vi "Life Support.vi"() -> ()   [LabVIEW 2020]
uses:
  <vilib>/regexp/Match Regular Expression.xnode
panel:
  out "Life Support":u32
  out "CO2":u32
  out "O2":u32
  in  "Input":string="110011110101\n110011100010\n010100011010\n011001100000\n010011011101\n011110111000\n111111000100\n000100010001\n101101010011\n100101101100\n001111011010\n011111111101\n010111000000\n000011101000\n100101010010\n010011000010\n000011000000\n111100110010\n100100101110\n110000110100\n011110010000\n010101000000\n001000110001\n010111000100\n110111010100\n011001110110\n110001001101\n001101010010\n110111110100\n100111110111\n001001110010\n001100011111\n001111110010\n100111000111\n101111100001\n011100001100\n000000000111\n101111110001\n110111001101\n101111011010\n100101001111\n011101111111\n101101010101\n011011111000\n011100101001\n001101010100\n00..."
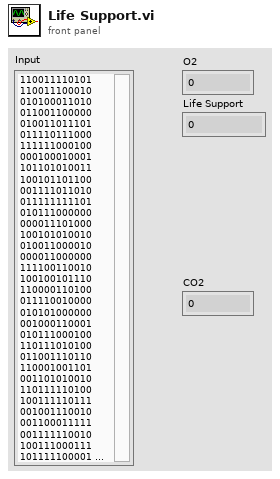
[diagram p1: front panel]
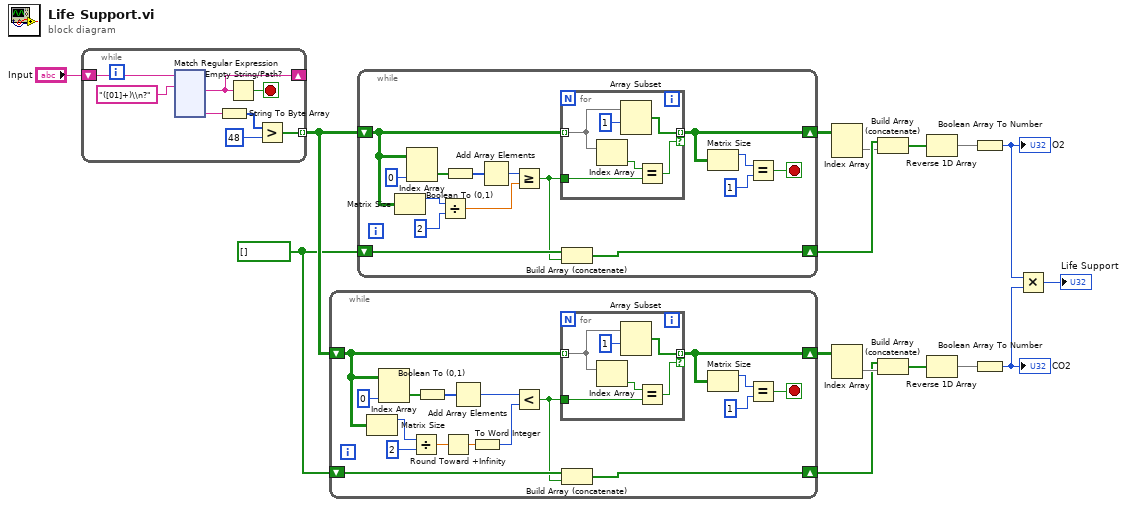
[diagram p0: block diagram]
diagram:
  w4 = bool[] []
  n1 = while {
    shift-right: [w22] -> _
    shift-left: "Input" -> [w24]
    tunnel: [w17] -> w5 mode=indexing
    stop <- w21 stop-if-true
    n2 = xnode "Match Regular Expression"("input string"=w24, "regular expression"="([01]+)\\n?") -> ("after match"=w22:string, "submatch 1"=w20:string)  [unwired: 4 in, 4 out]
    n3 = String To Byte Array(string=w20) -> (unsigned byte array=w19:u8[])
    n4 = Empty String/Path?(string/path=w22) -> (empty?=w21:bool)
    n5 = Greater?(x=w19, y=u8 48) -> (0:w17:bool[])
  }
  n6 = while {
    shift-right: [w150] -> w6
    shift-left: w4 -> [w152]
    shift-right: [w149] -> w7
    shift-left: w5 -> [w153]
    stop <- w147 stop-if-true
    n7 = Matrix Size(0:w153) -> (1:w145:i32)  [unwired: 1 out]
    n8 = Index Array(array=w153, index (col)=0 ("disabled index (col)")) -> (element=w156:bool[])  [unwired: 1 in]
    n9 = Divide(x=w145, y=2) -> (x/y=w143:dbl)
    n10 = Boolean To (0,1)(Boolean=w156) -> (0, 1=w155:i16[])
    n11 = Round Toward +Infinity(x=w143) -> (ceil(x): smallest int >= x=w142:dbl)
    n12 = Add Array Elements(numeric array=w155) -> (sum=w154:i16)
    n13 = To Word Integer(number=w142) -> (16bit integer=w141:i16)
    n14 = Less?(x=w154, y=w141) -> (x < y?=w151:bool)
    n15 = for {
      tunnel: w153 -> [w161] mode=indexing
      tunnel: w151 -> [w163]
      tunnel: [w159] -> w149 mode=indexing if=w158
      n16 = Index Array(array=w161) -> (element=w162:bool)  [unwired: 1 in]
      n17 = Array Subset(array=w161, index=1) -> (w159:bool[])  [unwired: 1 in]
      n18 = Equal?(x=w162, y=w163) -> (x = y?=w158:bool)
    }
    n19 = Build Array (concatenate)(w152, w151) -> (w150:bool[])
    n20 = Matrix Size(0:w149) -> (1:w146:i32)  [unwired: 1 out]
    n21 = Equal?(x=w146, y=1) -> (x = y?=w147:bool)
  }
  n22 = while {
    shift-right: [w171] -> w15
    shift-left: w4 -> [w173]
    shift-right: [w170] -> w14
    shift-left: w5 -> [w174]
    stop <- w168 stop-if-true
    n23 = Matrix Size(0:w174) -> (1:w166:i32)  [unwired: 1 out]
    n24 = Index Array(array=w174, index (col)=0 ("disabled index (col)")) -> (element=w177:bool[])  [unwired: 1 in]
    n25 = Divide(x=w166, y=2) -> (x/y=w164:dbl)
    n26 = Boolean To (0,1)(Boolean=w177) -> (0, 1=w176:i16[])
    n27 = Add Array Elements(numeric array=w176) -> (sum=w175:i16)
    n28 = Greater Or Equal?(x=w175, y=w164) -> (x >= y?=w172:bool)
    n29 = for {
      tunnel: w174 -> [w182] mode=indexing
      tunnel: w172 -> [w184]
      tunnel: [w180] -> w170 mode=indexing if=w179
      n30 = Index Array(array=w182) -> (element=w183:bool)  [unwired: 1 in]
      n31 = Array Subset(array=w182, index=1) -> (w180:bool[])  [unwired: 1 in]
      n32 = Equal?(x=w183, y=w184) -> (x = y?=w179:bool)
    }
    n33 = Build Array (concatenate)(w173, w172) -> (w171:bool[])
    n34 = Matrix Size(0:w170) -> (1:w167:i32)  [unwired: 1 out]
    n35 = Equal?(x=w167, y=1) -> (x = y?=w168:bool)
  }
  n36 = Index Array(array=w14) -> (element=w13:bool[])  [unwired: 2 in]
  n37 = Index Array(array=w7) -> (element=w8:bool[])  [unwired: 2 in]
  n38 = Build Array (concatenate)(w15, w13) -> (w12:bool[])
  n39 = Build Array (concatenate)(w6, w8) -> (w9:bool[])
  n40 = Reverse 1D Array(array=w12) -> (reversed array=w11:bool[])
  n41 = Reverse 1D Array(array=w9) -> (reversed array=w10:bool[])
  n42 = Boolean Array To Number(Boolean array=w11) -> (number=w3:u32)
  "O2" <- w3
  n43 = Boolean Array To Number(Boolean array=w10) -> (number=w2:u32)
  "CO2" <- w2
  n44 = Multiply(x=w3, y=w2) -> (x*y=→"Life Support":u32)
